vi "10nov_TEST.vi"() -> ()   [LabVIEW 2020]
uses:
  <instrlib>/Agilent B2900 Series/Agilent B2900 Series.lvlib
panel:
  out "I":dbl
  out "R":dbl
  out "V":dbl
  in  "VISA resource name":refnum<visa-resource-name>="USB0::0x0957::0x8E18::MY51140695::INSTR"
  in  "Source Voltage(V)":dbl
  in  "Channel":u32(ring) items=["Not Selected", "1", "2"]
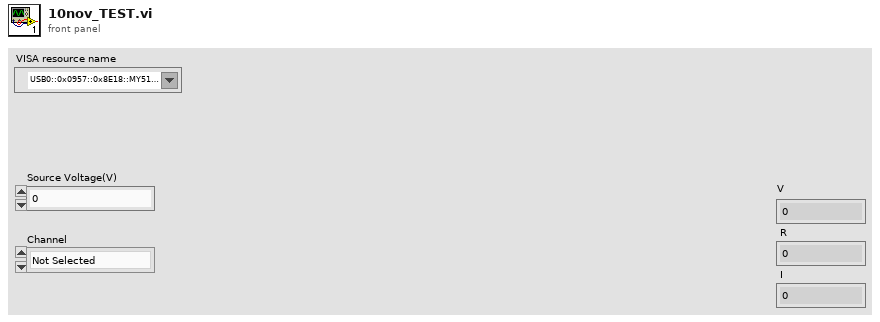
[diagram p1: front panel]
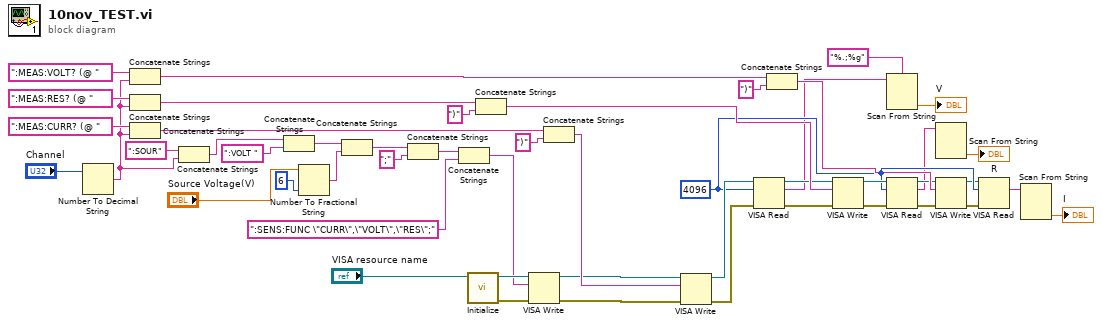
[diagram p0: block diagram]
diagram:
  w16 = u32 4096 ("byte count")
  n1 = Number To Decimal String(number="Channel") -> (decimal integer string=w21:string)  [unwired: 1 in]
  n2 = Concatenate Strings(":MEAS:VOLT? (@ " ("string"), w21) -> (w29:string)
  n3 = Concatenate Strings(":MEAS:RES? (@ " ("string"), w21) -> (w25:string)
  n4 = Concatenate Strings(":MEAS:CURR? (@ " ("string"), w21) -> (w33:string)
  n5 = Concatenate Strings(":SOUR", w21) -> (w48:string)
  n6 = Concatenate Strings(w48, ":VOLT ") -> (w46:string)
  n7 = Number To Fractional String(number="Source Voltage(V)", precision (6)=i16 6) -> (F-format string=w41:string)  [unwired: 2 in]
  n8 = Concatenate Strings(w46, w41) -> (w45:string)
  n9 = Concatenate Strings(w45, ";" ("string")) -> (w40:string)
  n10 = Concatenate Strings(w40, ":SENS:FUNC \"CURR\",\"VOLT\",\"RES\";") -> (w34:string)
  n11 = call <instrlib>:"Initialize.vi"("VISA resource name"="VISA resource name") -> ("error out"=w35:errorcluster, "VISA resource name out"=w36:refnum<visa-resource-name>)  [unwired: 9 in]
  n12 = Concatenate Strings(w25, ")" ("string")) -> (w22:string)
  n13 = VISA Write(VISA resource name=w36, write buffer=w34, error in (no error)=w35) -> (VISA resource name out=w8:refnum<visa-resource-name>, error out=w15:errorcluster)  [unwired: 1 out]
  n14 = Concatenate Strings(w33, ")" ("string")) -> (w30:string)
  n15 = VISA Write(VISA resource name=w8, write buffer=w30, error in (no error)=w15) -> (VISA resource name out=w20:refnum<visa-resource-name>, error out=w19:errorcluster)  [unwired: 1 out]
  n16 = VISA Read(VISA resource name=w20, byte count=w16, error in (no error)=w19) -> (VISA resource name out=w14:refnum<visa-resource-name>, read buffer=w1:string, error out=w13:errorcluster)  [unwired: 1 out]
  n17 = Concatenate Strings(w29, ")" ("string")) -> (w26:string)
  n18 = VISA Write(VISA resource name=w14, write buffer=w22, error in (no error)=w13) -> (VISA resource name out=w18:refnum<visa-resource-name>, error out=w17:errorcluster)  [unwired: 1 out]
  n19 = Scan From String(format string="%.;%g", input string=w1) -> (output 1=→"V":dbl)  [unwired: 3 in, 3 out]
  n20 = VISA Read(VISA resource name=w18, byte count=w16, error in (no error)=w17) -> (VISA resource name out=w12:refnum<visa-resource-name>, read buffer=w5:string, error out=w11:errorcluster)  [unwired: 1 out]
  n21 = Scan From String(input string=w5) -> (output 1=→"R":dbl)  [unwired: 4 in, 3 out]
  n22 = VISA Write(VISA resource name=w12, write buffer=w26, error in (no error)=w11) -> (VISA resource name out=w10:refnum<visa-resource-name>, error out=w9:errorcluster)  [unwired: 1 out]
  n23 = VISA Read(VISA resource name=w10, byte count=w16, error in (no error)=w9) -> (read buffer=w4:string)  [unwired: 3 out]
  n24 = Scan From String(input string=w4) -> (output 1=→"I":dbl)  [unwired: 4 in, 3 out]
